vi "Write Handle.vi"(8 "error in":errorcluster, 10 "Session Handle":T1, 11 "Configurable Device in":refnum<class "Configurable Device.lvclass">) -> (0 "error out":errorcluster, 3 "Configurable Device out":refnum<class "Configurable Device.lvclass">)   [LabVIEW 2018, in "Device.lvlib" / "Configurable Device.lvclass"]
uses:
  Configurable Device.lvclass
  reusable/Session APIs/File Access/Config Data/Config Session.ctl
  reusable/Session APIs/File Access/Config Data/Config Data.lvclass
  Configurable Device.lvclass/Configurable Device.ctl
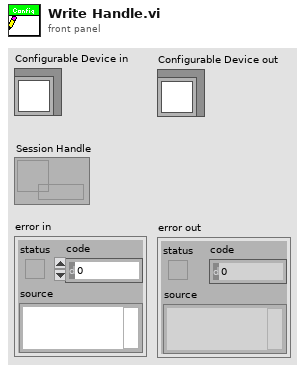
[diagram p1: front panel]
types:
  T1 = typedef "Config Data.lvclass/Config Session.ctl" = refnum<data-value>
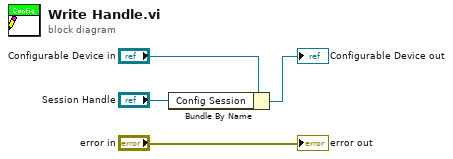
[diagram p0: block diagram]
diagram:
  n1 = Bundle By Name(cluster="Configurable Device in", "Config Session"="Session Handle") -> (→"Configurable Device out":refnum<class "Configurable Device.lvclass">)
  "error out" <- "error in"
